vi "Create YIELD msg.vi"(8 "error in (no error)":errorcluster, 11 "Yield request":T1) -> (0 "error out":errorcluster, 3 "String":string)   [LabVIEW 2020, in "wamplv.lvlib" / "WAMP Client.lvclass"]
uses:
  WAMP Client.lvclass
  TypeDef/YIELD request data.ctl
  TypeDef/WAMP Message Codes.ctl
  WAMP Client.lvclass/WAMP Client.ctl
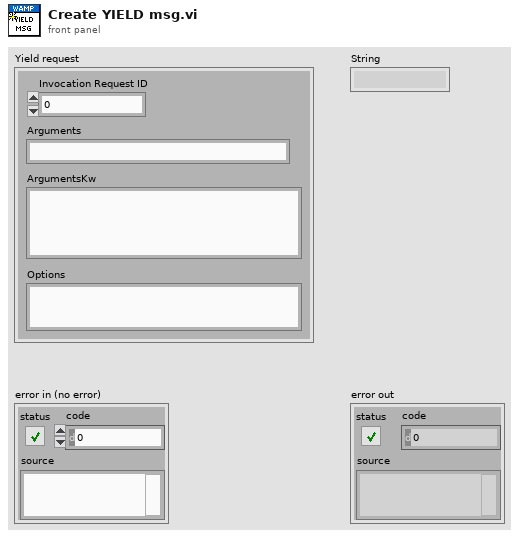
[diagram p1: front panel]
types:
  T1 = typedef "wamplv.lvlib/WAMP Client.lvclass/YIELD request data.ctl" = cluster{"Invocation Request ID":u64, "Arguments":string, "ArgumentsKw":string, "Options":string}
  T2 = typedef "wamplv.lvlib/WAMP Client.lvclass/WAMP Message Codes.ctl" = u16
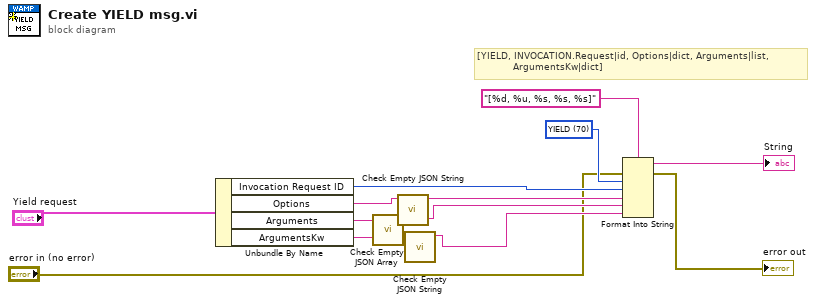
[diagram p0: block diagram]
diagram:
  w5 = T2 70 items=["HELLO"=1, "WELCOME"=2, "ABORT"=3, "GOODBYE"=6, "ERROR"=8, "PUBLISH"=16, "PUBLISHED"=17, "SUBSCRIBE"=32, "SUBSCRIBED"=33, "UNSUBSCRIBE"=34, "UNSUBSCRIBED"=35, "EVENT"=36, "CALL"=48, "RESULT"=59, "REGISTER"=64, "REGISTERED"=65, "UNREGISTER"=66, "UNREGISTERED"=67, "INVOCATION"=68, "YIELD"=70] ("Message Codes")
  # "[YIELD, INVOCATION.Request|id, Options|dict, Arguments|list,\n            ArgumentsKw|dict]"
  n1 = Unbundle By Name("Yield request") -> ("Invocation Request ID"=w7:u64, "Options"=w10:string, "Arguments"=w13:string, "ArgumentsKw"=w8:string)
  n2 = call "Check Empty JSON Array.vi"("JSON"=w13) -> ("JSON"=w12:string)  [unwired: 10 in]
  n3 = call "Check Empty JSON String.vi"("JSON"=w10) -> ("JSON"=w11:string)  [unwired: 10 in]
  n4 = call "Check Empty JSON String.vi"("JSON"=w8) -> ("JSON"=w9:string)  [unwired: 10 in]
  n5 = Format Into String(format string="[%d, %u, %s, %s, %s]" ("element"), error in="error in (no error)", w5, w7, w11, w12, w9) -> (resulting string=→"String":string, error out=→"error out":errorcluster)  [unwired: 1 in]
